vi "LJUD_ErrorToString.vi"(8 "error in":errorcluster) -> (2 "String":string)   [LabVIEW 2021]
doc: "ErrorToString converts a numeric errorcode\nto a string version of the error.\n\n6000 is added to all LabJack errorcodes to put them\nin the 5000-9999 range."
uses:
  labjackud.dll
panel:
  # "ErrorToString converts a numeric errorcode\nto a string version of the error.\n\n6000 is added to all LabJack errorcodes to put them\nin the 5000-9999 range."
  # "6000 is added to all LabJack Errorcodes to put them in the 5000-9999 range."
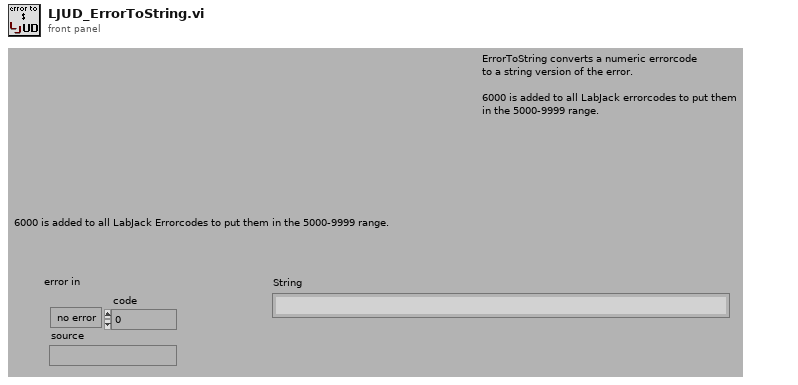
[diagram p1: front panel]
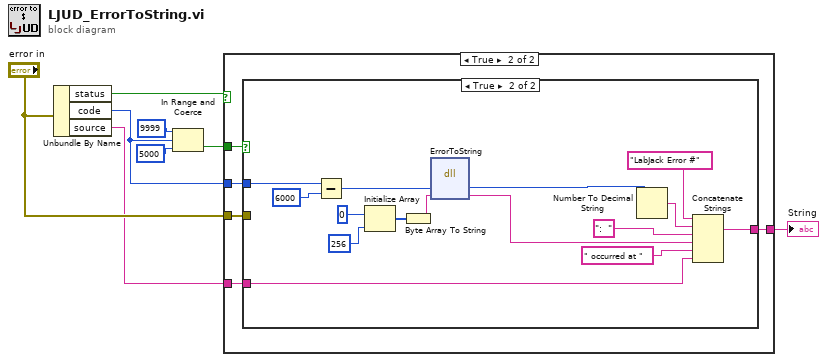
[diagram p0: block diagram]
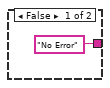
[diagram p2: hidden frame]
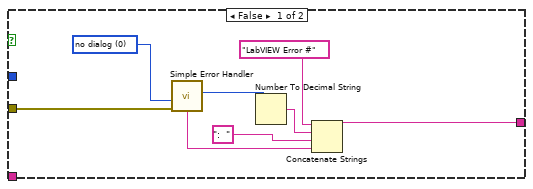
[diagram p3: hidden frame]
diagram:
  n1 = Unbundle By Name("error in") -> ("status"=w1:bool, "code"=w2:i32, "source"=w4:string)
  n2 = In Range and Coerce(upper limit=9999, x=w2, lower limit=5000) -> (In Range?=w6:bool)  [unwired: 1 out]
  n3 = case shown="True" w1 {
    tunnel: ["No Error" w14] -> w8
    tunnel: w6 -> [_ w13]
    tunnel: w2 -> [_ w12]
    tunnel: "error in" -> [_ w11]
    tunnel: w4 -> [_ w10]
    frame False {
    }
    frame True {
      n4 = case shown="True" w13 {
        tunnel: [w15 w24] -> w14
        tunnel: w12 -> [_ w33]
        tunnel: w11 -> [w21 _]
        tunnel: w10 -> [_ w25]
        frame False {
          w22 = u16 0 items=["no dialog", "OK message", "continue or stop message"] ("type of dialog (OK msg:1)")
          n5 = call <vilib>:"Simple Error Handler.vi"("type of dialog (OK msg:1)"=w22, "error in (no error)"=w21) -> ("code out"=w18:i32, "message"=w20:string)  [unwired: 3 in, 3 out]
          n6 = Number To Decimal String(number=w18) -> (decimal integer string=w17:string)  [unwired: 1 in]
          n7 = Concatenate Strings("LabVIEW Error #" ("Substring"), w17, ":  " ("Substring"), w20) -> (w15:string)
        }
        frame True {
          n8 = Subtract(x=w33, y=6000) -> (x-y=w32:i32)
          n9 = Initialize Array(u8 0 ("Element Data"), 256 ("Dimension Size")) -> (w35:u8[])
          n10 = Byte Array To String(unsigned byte array=w35) -> (string=w34:string)
          n11 = dll-call lib="labjackud.dll" fn="ErrorToString"("ErrorCode"=w32, "String"=w34) -> ("ErrorCode"=w28:i32, "String"=w27:string)  [unwired: 4 in, 2 out]
          n12 = Number To Decimal String(number=w28) -> (decimal integer string=w30:string)  [unwired: 1 in]
          n13 = Concatenate Strings("LabJack Error #" ("Substring"), w30, ":  " ("Substring"), w27, " occurred at " ("Substring"), w25) -> (w24:string)
        }
      }
    }
  }
  "String" <- w8
